vi "Path as UTF-8 Path (UTF-8 Path).vi"(6 "error in":errorcluster, 9 "Path":refnum<class "UTF-8 Path.lvclass">) -> (1 "UTF-8 Path":refnum<class "UTF-8 Path.lvclass">, 4 "error out":errorcluster)   [LabVIEW 2020, in "G-Unicode.lvlib"]
doc: "Converts the input path to a UTF-8 Path. Valid inputs are a UTF-8 Path class, or LabVIEW path."
uses:
  G-Unicode.lvlib
  Types/UTF-8 Path/UTF-8 Path.lvclass
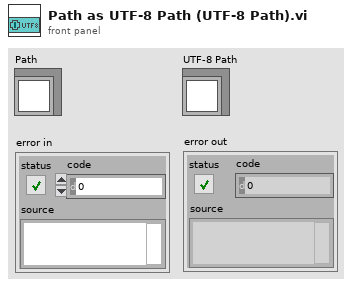
[diagram p1: front panel]
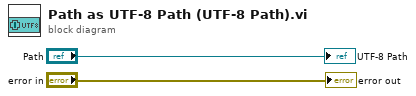
[diagram p0: block diagram]
diagram:
  "UTF-8 Path" <- "Path"
  "error out" <- "error in"
